vi "DSF.Execution.Runtime.Plugin Manager.Get Plugins.vi"(8 "error in (no error)":errorcluster, 11 "Plugin Manager in":refnum<class "DSF.Engine.Runtime.Plugin Manager.lvclass">) -> (0 "error out":errorcluster, 2 "Plugins":refnum<class "DSF.Engine.Plugin.Runtime.lvclass">[](array[class]), 3 "Plugin Manager out":refnum<class "DSF.Engine.Runtime.Plugin Manager.lvclass">)   [LabVIEW 2016, in "DSF.Engine.lvlib" / "DSF.Engine.Runtime.Plugin Manager.lvclass"]
uses:
  DSF.Engine.Runtime.Plugin Manager.lvclass
  Plugin/DSF.Engine.Plugin.Runtime.lvclass
  DSF.Engine.Runtime.Plugin Manager.lvclass/DSF.Engine.Runtime.Plugin Manager.ctl
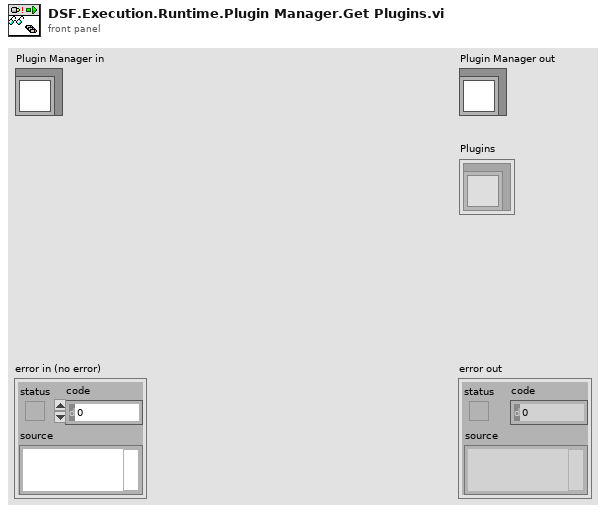
[diagram p1: front panel]
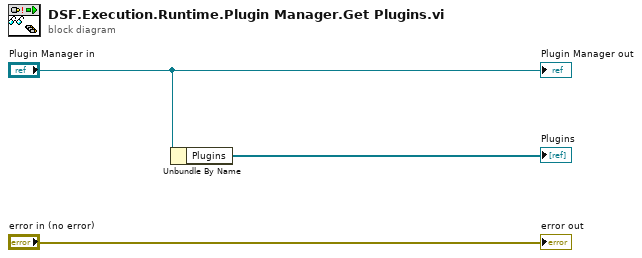
[diagram p0: block diagram]
diagram:
  n1 = Unbundle By Name("Plugin Manager in") -> ("Plugins"=→"Plugins":refnum<class "DSF.Engine.Plugin.Runtime.lvclass">[])
  "error out" <- "error in (no error)"
  "Plugin Manager out" <- "Plugin Manager in"
